vi "GUNSC_LibOpen.vi"(8 "error in (no error)":errorcluster, 10 "libpath":string) -> (0 "error out":errorcluster, 2 "return value":i32)   [LabVIEW 2014]
uses:
  public/c/lib/libunsc.so
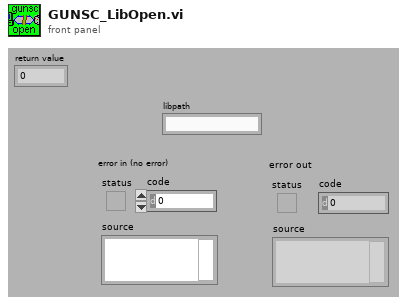
[diagram p1: front panel]
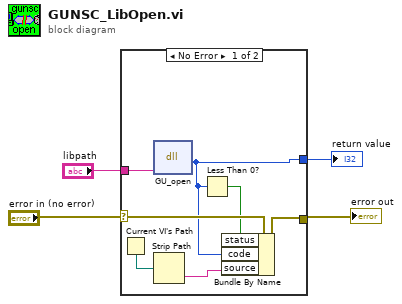
[diagram p0: block diagram]
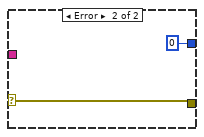
[diagram p2: hidden frame]
diagram:
  n1 = case shown="No Error" "error in (no error)" {
    selector: "error in (no error)" -> [w11 w13]
    tunnel: [w9 0] -> w4
    tunnel: [w6 w13] -> w2
    tunnel: "libpath" -> [w5 _]
    frame No Error {
      n2 = Current VI's Path() -> (path=w8:path)
      n3 = dll-call lib="home/sispi/Panview-1.13.0-64b/PAN/Modules/GUNSC/public/c/lib/libunsc.so" fn="GU_open"("libpath"=w5) -> (w9:i32)  [unwired: 4 in, 2 out]
      n4 = Strip Path(path=w8) -> (name=w7:string)  [unwired: 1 out]
      n5 = Less Than 0?(x=w9) -> (x < 0?=w10:bool)
      n6 = Bundle By Name(cluster=w11, "status"=w10, "code"=w9, "source"=w7) -> (w6:errorcluster)
    }
    frame Error {
    }
  }
  "return value" <- w4
  "error out" <- w2
